vi "Selected Channel Read.vi"(4 "error in (no error)":errorcluster, 6 "Container State":T5, 7 "Display State In":T2={"Hierarchy"=[], "File/Directory Path"=path "", "Relative File Paths"=[], "Hide Undefined Channels"=FALSE, "Static File Structure"=FALSE, "Filtering"={"Filtered Groups"=[], "Group Filter Mode"=enum."Exclude", "Group Filter Regex?"=FALSE, "Filtered Channels"=[], "Channel Filter Mode"=enum."Exclude", "Channel Filter Regex?"=FALSE, "Filter Time Start"=timestamp(0 s since 1904-01-01), "Filter Time End"=timestamp(0 s since 1904-01-01), "Time Filter Mode"=enum."Include", "Time Filter Enabled"=FALSE}, "File Contents Tree"=refnum, "Properties Table"=refnum, "Loading Indicator"=refnum}) -> (0 "error out":errorcluster, 2 "Value":T1[](array[typedef]), 3 "Display State Out":T2={"Hierarchy"=[], "File/Directory Path"=path "", "Relative File Paths"=[], "Hide Undefined Channels"=FALSE, "Static File Structure"=FALSE, "Filtering"={"Filtered Groups"=[], "Group Filter Mode"=enum."Exclude", "Group Filter Regex?"=FALSE, "Filtered Channels"=[], "Channel Filter Mode"=enum."Exclude", "Channel Filter Regex?"=FALSE, "Filter Time Start"=timestamp(0 s since 1904-01-01), "Filter Time End"=timestamp(0 s since 1904-01-01), "Time Filter Mode"=enum."Include", "Time Filter Enabled"=FALSE}, "File Contents Tree"=refnum, "Properties Table"=refnum, "Loading Indicator"=refnum})   [LabVIEW 2017, in "XTree.xctl"]
doc: "Gets the channel info from whatever is selected in the tree. If something at a higher level in the hierarchy than channels is selected, all of the channels underneath will be given."
uses:
  <vilib>/addons/_NIFileIO/XTree/XTree.xctl
  <vilib>/_xctls/Container State.ctl
  <vilib>/addons/_NIFileIO/XTree/State.ctl
  <vilib>/addons/_NIFileIO/XTree/Controls/Filter Settings.ctl
  <vilib>/addons/_NIFileIO/XTree/Controls/Filter Mode.ctl
  <vilib>/addons/_NIFileIO/XTree/Controls/Tree Selection Data.ctl
  <vilib>/_xctls/XControlSupport.lvlib
panel:
  # "Replace the Value Indicator below with an Indicator of desired type.\nDo not remove this Indicator or the others from the connector pane. \nDo not change the connector pane pattern.\nThe Value Indicator should always be the second terminal from top on the output side in the connector pane."
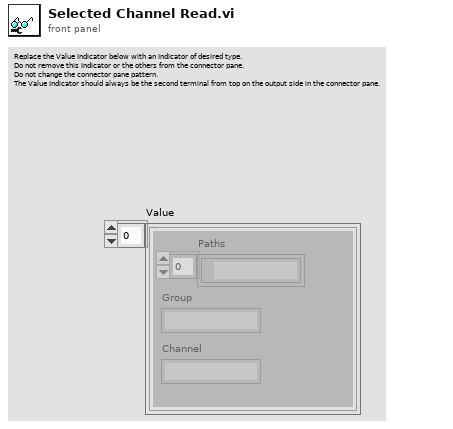
[diagram p1: front panel]
types:
  T1 = typedef "XTree.xctl/Tree Selection Data.ctl" = cluster{"Paths":path[], "Group":string, "Channel":string}
  T2 = typedef "XTree.xctl/State.ctl" = cluster{"Hierarchy":string[], "File/Directory Path":path, "Relative File Paths":string[], "Hide Undefined Channels":bool, "Static File Structure":bool, "Filtering":T3, "File Contents Tree":refnum<vi>, "Properties Table":refnum<vi>, "Loading Indicator":refnum<vi>}
  T3 = typedef "XTree.xctl/Filter Settings.ctl" = cluster{"Filtered Groups":string[], "Group Filter Mode":T4, "Group Filter Regex?":bool, "Filtered Channels":string[], "Channel Filter Mode":T4, "Channel Filter Regex?":bool, "Filter Time Start":timestamp, "Filter Time End":timestamp, "Time Filter Mode":T4, "Time Filter Enabled":bool}
  T4 = typedef "XTree.xctl/Filter Mode.ctl" = enum16{"Exclude", "Include"}
  T5 = typedef "XControlSupport.lvlib/Container State.ctl" = cluster{"Indicator?":bool, "Run Mode?":bool, " Refnum":refnum<vi>}
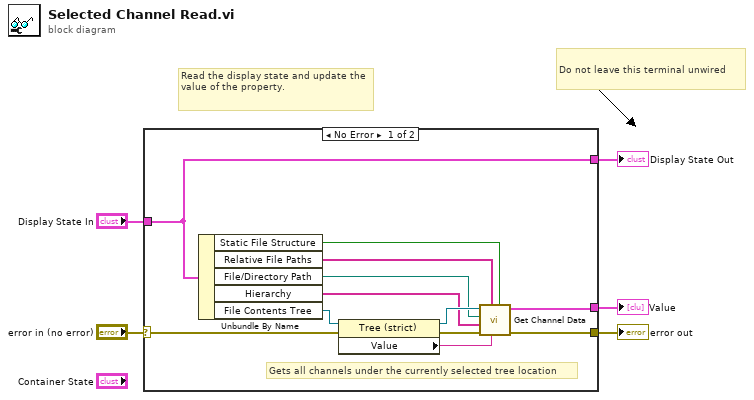
[diagram p0: block diagram]
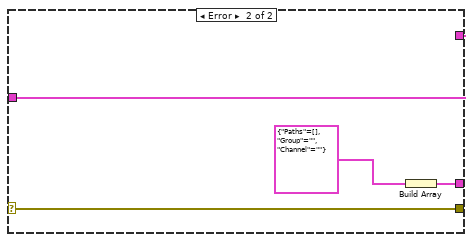
[diagram p2: hidden frame]
diagram:
  # "Read the display state and update the value of the property."
  # "Do not leave this terminal unwired"
  n1 = case shown="No Error" "error in (no error)" {
    selector: "error in (no error)" -> [w14 w20]
    tunnel: "Display State In" -> [w15 w21]
    tunnel: [w16 w20] -> w4
    tunnel: [w15 w21] -> w3
    tunnel: [w13 w18] -> w1
    frame No Error {
      # "Gets all channels under the currently selected tree location"
      n2 = Unbundle By Name(w15) -> ("Static File Structure"=w10:bool, "Relative File Paths"=w11:string[], "File/Directory Path"=w8:path, "Hierarchy"=w7:string[], "File Contents Tree"=w12:refnum<vi>)
      n3 = property class="Tree (strict)"(reference=w12, error in=w14) -> (reference out=w9:refnum<vi>, error out=w17:errorcluster, "Value"=w6:string)
      n4 = call <vilib>:"Get Channel Data.vi"("Static File Structure"=w10, "Tree Location"=w6, "Relative File Paths"=w11, "error in (no error)"=w17, "Hierarchy"=w7, "Data Directory"=w8, "TreeControl in"=w9) -> ("error out"=w16:errorcluster, "Tree Selection Data Array"=w13:T1[])  [unwired: 3 in]
    }
    frame Error {
      n5 = Build Array(T1 {"Paths"=[], "Group"="", "Channel"=""} ("Tree Selection Data")) -> (w18:T1[])
    }
  }
  "error out" <- w4
  "Display State Out" <- w3
  "Value" <- w1
